vi "Acknowledge.vi"(8 "error in (no error)":errorcluster, 10 "Message in":refnum<class "AcknowledgeMessage.lvclass">, 11 "Galvo in":refnum<class "ImagingModeSPIM.lvclass">) -> (0 "error out":errorcluster, 3 "Galvo out":refnum<class "ImagingModeSPIM.lvclass">)   [LabVIEW 2012, in "ImagingModeSPIM.lvclass"]
doc: "The acknowledge method processes the command 'acknowledge'. \n\nWhen a message is sent that requires that the component responds with a confirmation of reception, the 'acknowledge' command should be used."
uses:
  ImagingModeSPIM.lvclass
  <vilib>/Distrio/Murmex/AcknowledgeMessage/AcknowledgeMessage.lvclass
  <vilib>/Distrio/Murmex/Murmex/Murmex.lvclass
panel:
  # "This method is called when the ACKNOWLEDGE\ntrigger is sent. \n\nOverride this method when your component needs to\nrespond to this trigger. \n\nCall parent for proper implementation"
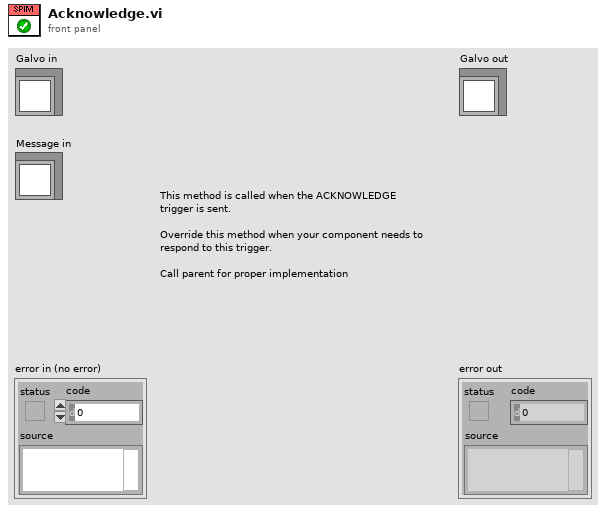
[diagram p1: front panel]
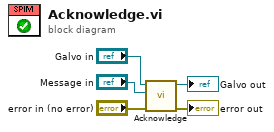
[diagram p0: block diagram]
diagram:
  n1 = call-parent "Acknowledge.vi"("error in (no error)"="error in (no error)", "Message in"="Message in", "Murmex in"="Galvo in") -> ("error out"=→"error out":errorcluster, "Murmex out"=→"Galvo out":refnum<class "ImagingModeSPIM.lvclass">)  [unwired: 7 in]
